vi "Display.vi"() -> ()   [LabVIEW 2018]
panel:
  out "Degrees C":dbl
  in  "Stop (F)":bool
  out "Waveform Chart C":dbl(graph)=-97179394.32439524
  out "Waveform Chart F":dbl(graph)=-174922877.78391144
  out "Degrees F":dbl
  in  "CJC Offset":dbl
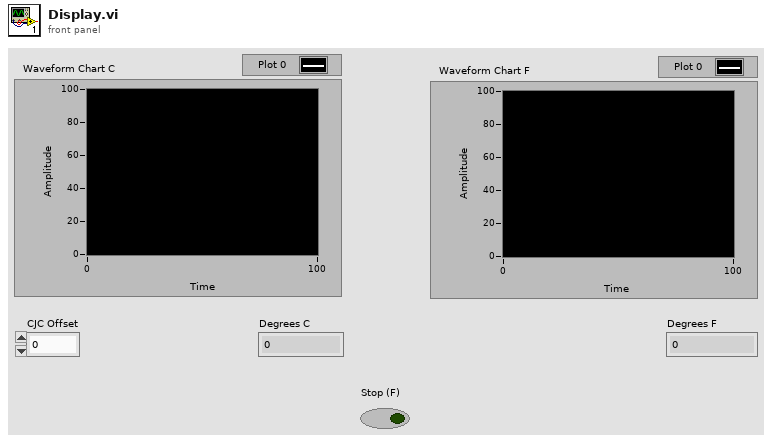
[diagram p1: front panel]
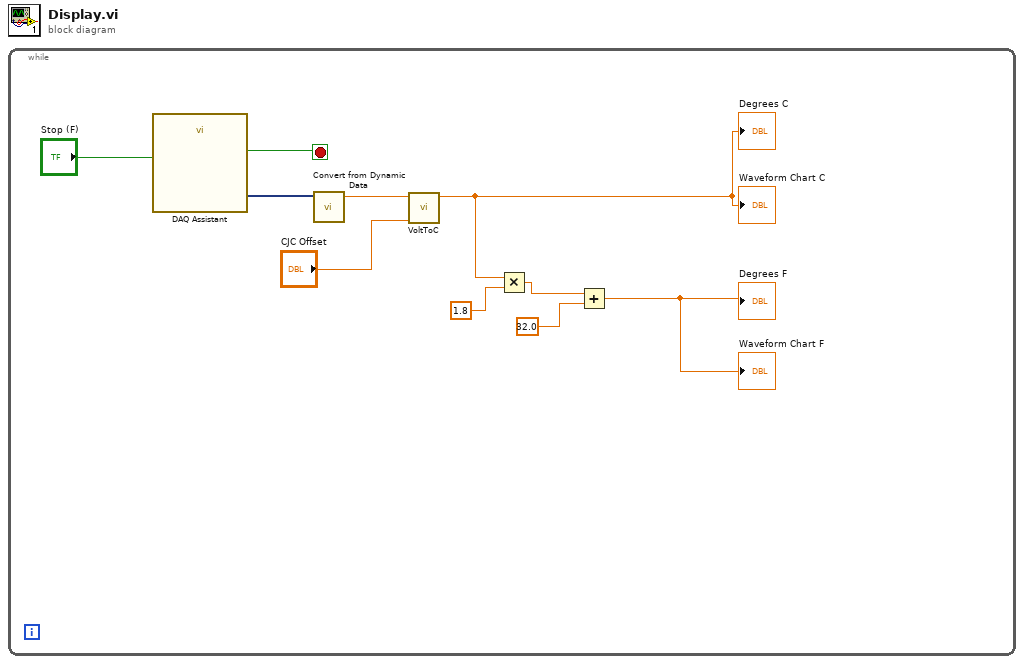
[diagram p0: block diagram]
diagram:
  n1 = while {
    stop <- w3 stop-if-true
    n2 = call "DAQ Assistant"("stop (F)"="Stop (F)") -> ("data"=w2:dynamicdata, "stopped"=w3:bool)  [unwired: 15 in, 2 out]
    n3 = call "Convert from Dynamic Data"("Dynamic Data Type"=w2) -> ("Scalar"=w1:dbl)  [unwired: 3 in]
    n4 = call "VoltToC.vi"("Offset"="CJC Offset", "Thermoelectric Voltage"=w1) -> ("Degrees C"=w5:dbl)  [unwired: 9 in]
    "Waveform Chart C" <- w5
    "Degrees C" <- w5
    n5 = Multiply(x=w5, y=1.8) -> (x*y=w8:dbl)
    n6 = Add(x=w8, y=32.0) -> (x+y=→"Degrees F" →"Waveform Chart F":dbl)
  }
